vi "Configure Serial Bus (SENT - Trigger).vi"(0 "VISA resource name":refnum<visa-resource-name>, 1 "Slow Data (-1)":i32=-1, 2 "Tolerance (1)":i32=1, 5 "Serial Bus Name (1: Serial Bus 1)":u16(ring)=1 items=["Serial Bus 1"=1, "Serial Bus 2"=2], 7 "Trigger Type\n(0: Start of Fast Channel Message)":u16(ring) items=["Start of Fast Channel Message", "Start of Slow Channel Message", "Fast Channel SC & Data", "Slow Channel Message ID", "Slow Channel Message ID & Data", "Tolerance Violation", "Fast Channel CRC error", "Slow Channel CRC error", "All CRC errors", "Pulse Period Error", "Successive Sync Pulses Error (1/64)"], 9 "Fast Data (\"0\")":string="\"0\"", 11 "error in (no error)":errorcluster, 12 "Slow Length (0: Short)":u16(ring) items=["Short", "Long"], 13 "Slow ID (-1)":i32=-1) -> (4 "VISA resource name out":refnum<visa-resource-name>, 15 "error out":errorcluster)   [LabVIEW 2017, in "Agilent 2000 3000 X-Series.lvlib"]
doc: "Configures SENT trigger properties.\n\nNote:\nThis VI is not supported by EDUX1052A/G, DSOX1202A/G, DSOX1204A/G models"
uses:
  Agilent 2000 3000 X-Series.lvlib
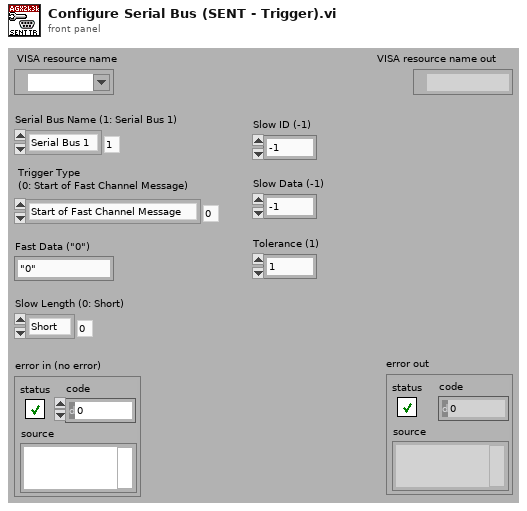
[diagram p1: front panel]
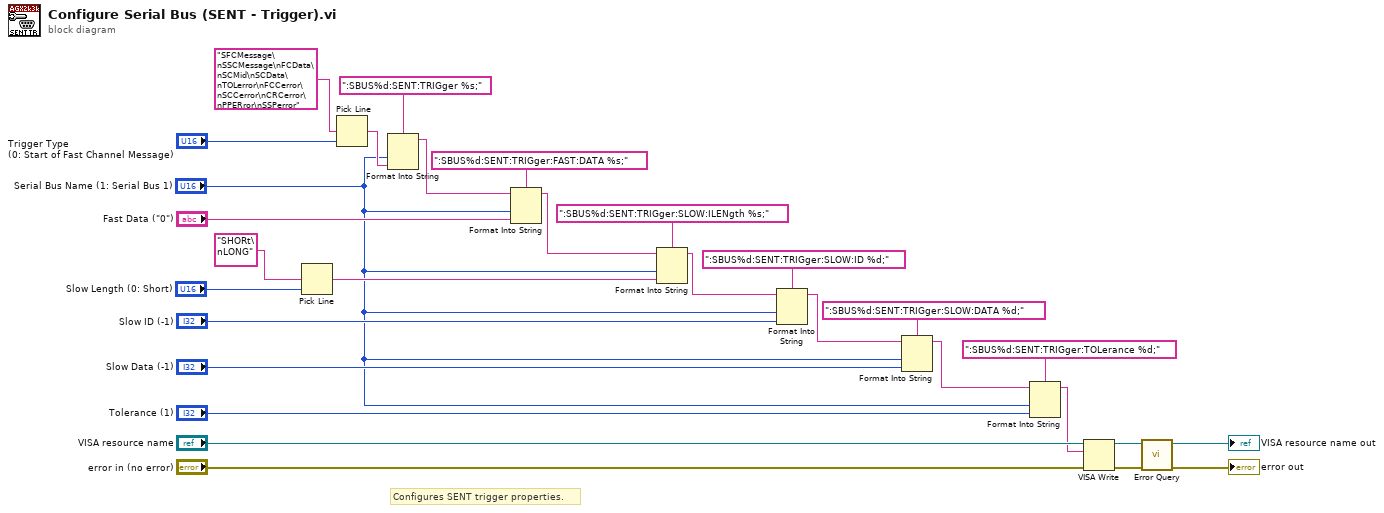
[diagram p0: block diagram]
diagram:
  # "Configures SENT trigger properties."
  n1 = Pick Line(multi-line string="SHORt\nLONG", line index="Slow Length (0: Short)") -> (output string=w21:string)  [unwired: 1 in]
  n2 = Pick Line(multi-line string="SFCMessage\nSSCMessage\nFCData\nSCMid\nSCData\nTOLerror\nFCCerror\nSCCerror\nCRCerror\nPPERror\nSSPerror", line index="Trigger Type\n(0: Start of Fast Channel Message)") -> (output string=w26:string)  [unwired: 1 in]
  n3 = Format Into String(format string=":SBUS%d:SENT:TRIGger %s;", "Serial Bus Name (1: Serial Bus 1)", w26) -> (resulting string=w19:string)  [unwired: 2 in, 1 out]
  n4 = Format Into String(format string=":SBUS%d:SENT:TRIGger:FAST:DATA %s;", initial string=w19, "Serial Bus Name (1: Serial Bus 1)", "Fast Data (\"0\")") -> (resulting string=w18:string)  [unwired: 1 in, 1 out]
  n5 = Format Into String(format string=":SBUS%d:SENT:TRIGger:SLOW:ILENgth %s;", initial string=w18, "Serial Bus Name (1: Serial Bus 1)", w21) -> (resulting string=w12:string)  [unwired: 1 in, 1 out]
  n6 = Format Into String(format string=":SBUS%d:SENT:TRIGger:SLOW:ID %d;", initial string=w12, "Serial Bus Name (1: Serial Bus 1)", "Slow ID (-1)") -> (resulting string=w11:string)  [unwired: 1 in, 1 out]
  n7 = Format Into String(format string=":SBUS%d:SENT:TRIGger:SLOW:DATA %d;", initial string=w11, "Serial Bus Name (1: Serial Bus 1)", "Slow Data (-1)") -> (resulting string=w10:string)  [unwired: 1 in, 1 out]
  n8 = Format Into String(format string=":SBUS%d:SENT:TRIGger:TOLerance %d;", initial string=w10, "Serial Bus Name (1: Serial Bus 1)", "Tolerance (1)") -> (resulting string=w5:string)  [unwired: 1 in, 1 out]
  n9 = VISA Write(VISA resource name="VISA resource name", write buffer=w5, error in (no error)="error in (no error)") -> (VISA resource name out=w3:refnum<visa-resource-name>, error out=w4:errorcluster)  [unwired: 1 out]
  n10 = call "Error Query.vi"("error in (no error)"=w4, "VISA resource name"=w3) -> ("error out"=→"error out":errorcluster, "VISA resource name out"=→"VISA resource name out":refnum<visa-resource-name>)  [unwired: 6 in, 2 out]
